vi "Chute.vi"() -> ()   [LabVIEW 2019]
uses:
  <vilib>/Rock Robotics/WPI/ThirdParty/Phoenix-LabVIEW/Motor Controller/Controls/CTRE_Phoenix_MotorControl_ControlMode.ctl
  <vilib>/Rock Robotics/WPI/Solenoid/WPI_SolenoidValue.ctl
  <vilib>/Rock Robotics/WPI/Utilities/WPI_GetSetVariantRefNum.vi
  <vilib>/Rock Robotics/WPI/Solenoid/WPI_SolenoidSetEnum.vi
  <vilib>/Rock Robotics/Network Tables/NT Write Boolean Array.vi
panel:
  in  "Control Mode 4":T1 items=["PercentOutput"=0, "Position"=1, "Velocity"=2, "Current"=3, "Follower"=5, "MotionProfile"=6, "MotionMagic"=7, "MotionProfileArc"=10, "Disabled"=15]
  in  "Control Mode 3":T1 items=["PercentOutput"=0, "Position"=1, "Velocity"=2, "Current"=3, "Follower"=5, "MotionProfile"=6, "MotionMagic"=7, "MotionProfileArc"=10, "Disabled"=15]
  in  "Control Mode 2":T1 items=["PercentOutput"=0, "Position"=1, "Velocity"=2, "Current"=3, "Follower"=5, "MotionProfile"=6, "MotionMagic"=7, "MotionProfileArc"=10, "Disabled"=15]
  in  "Control Mode":T1 items=["PercentOutput"=0, "Position"=1, "Velocity"=2, "Current"=3, "Follower"=5, "MotionProfile"=6, "MotionMagic"=7, "MotionProfileArc"=10, "Disabled"=15]
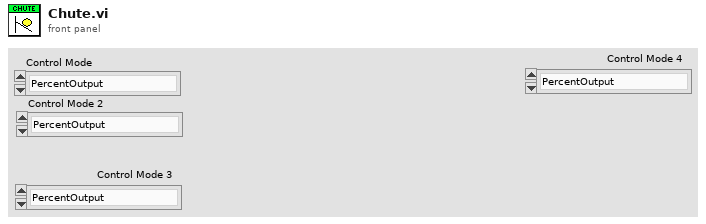
[diagram p1: front panel]
types:
  T1 = typedef "CTRE_Phoenix_MotorControl_ControlMode.ctl" = u16
  T2 = typedef "WPI_JoystickDevRef.ctl" = cluster{"Device":T3}
  T3 = typedef "WPI_JoystickDeviceEnum.ctl" = enum16{"USB 0", "USB 1", "USB 2", "USB 3", "USB 4", "USB 5"}
  T4 = typedef "WPI_SolenoidValue.ctl" = enum16{"Off", "On", "Forward", "Reverse"}
  T5 = typedef "WPI_SolenoidDevRef.ctl" = cluster{"DevStatus":errorcluster, "Pneumatics Control Module":u8, "Forward Solenoid Channel":T6, "Reverse Solenoid Channel":T6}
  T6 = typedef "WPI_SolenoidChannel.ctl" = enum8{"Solenoid 0", "Solenoid 1", "Solenoid 2", "Solenoid 3", "Solenoid 4", "Solenoid 5", "Solenoid 6", "Solenoid 7", "Invalid"}
  T7 = typedef "WPI_MotorControlDeviceRef.ctl" = cluster{"DeviceStatus":errorcluster, "Type":T8, "PWM":cluster{"PWM Channel":T9, "DeadBand":T10}, "CAN":cluster{"Device Number":u8, "SetOutput VI Ref":variant, "GetOutput VI Ref":variant, "Enable VI Ref":variant, "Disable VI Ref":variant, "Data":variant}, "Invert":bool, "DIO PWM":cluster{"PWM \"Enable\" Channel":T9, "DIOChannel":T11, "PWM Rate":dbl}}
  T8 = typedef "WPI_MotorControlType.ctl" = enum16{"PWM", "CAN", "DIO PWM"}
  T9 = typedef "FPGA_DIOPWMChannel.ctl" = enum8{"PWM 0", "PWM 1", "PWM 2", "PWM 3", "PWM 4", "PWM 5", "PWM 6", "PWM 7", "PWM 8", "PWM 9", "PWM MXP 0", "PWM MXP 1", "PWM MXP 2", "PWM MXP 3", "PWM MXP 4", "PWM MXP 5", "PWM MXP 6", "PWM MXP 7", "PWM MXP 8", "PWM MXP 9", "Invalid"}
  T10 = typedef "WPI_PWMDeadband.ctl" = cluster{"Name":string, "maxPositivePwm":i32, "minPositivePwm":i32, "centerPwm":i32, "maxNegativePwm":i32, "minNegativePwm":i32, "angularRange":u16}
  T11 = typedef "FPGA_DIOChannel.ctl" = enum8{"DIO 0", "DIO 1", "DIO 2", "DIO 3", "DIO 4", "DIO 5", "DIO 6", "DIO 7", "DIO 8", "DIO 9", "DIO MXP 0", "DIO MXP 1", "DIO MXP 2", "DIO MXP 3", "DIO MXP 4", "DIO MXP 5", "DIO MXP 6", "DIO MXP 7", "DIO MXP 8", "DIO MXP 9", "DIO MXP 10", "DIO MXP 11", "DIO MXP 12", "DIO MXP 13", "DIO MXP 14", "DIO MXP 15", "SPI Port CS1", "SPI Port CS2", "SPI Port CS3", "SPI Port MISO", "SPI Port MOSI", "Invalid"}
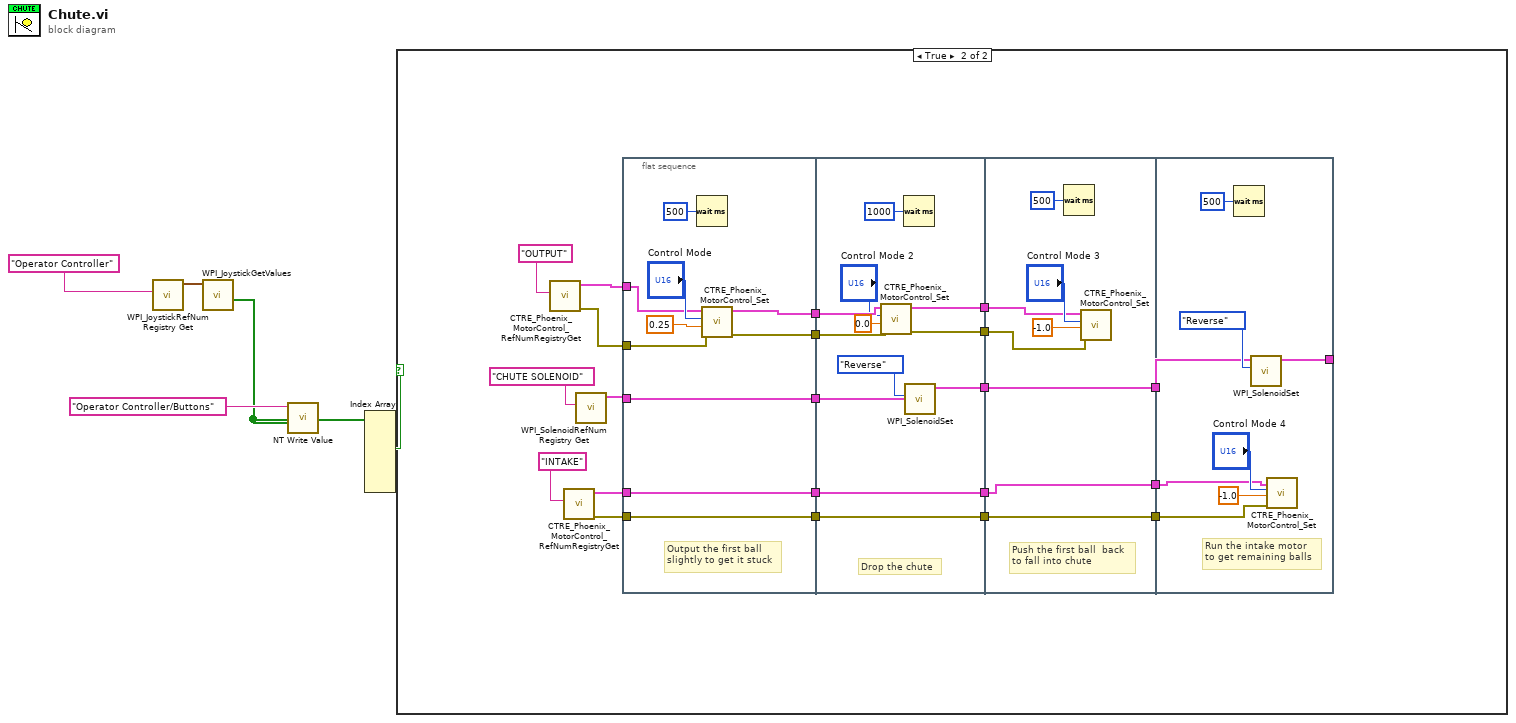
[diagram p0: block diagram]
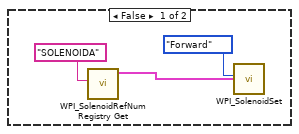
[diagram p2: hidden frame]
diagram:
  n1 = call <vilib>:"WPI_JoystickRefNum Registry Get.vi"("refnum name"="Operator Controller") -> ("JoystickDevRef"=w4:T2)  [unwired: 1 in, 9 out]
  n2 = call <vilib>:"WPI_JoystickGetValues.vi"("JoystickDevRef"=w4) -> ("Buttons"=w2:bool[])  [unwired: 6 in, 4 out]
  n3 = call-poly <vilib>:"NT Write Value.vi"("Boolean Array"=w2, "Name"="Operator Controller/Buttons") -> ()  [unwired: 9 in, 1 out]
  n4 = Index Array(array=w2) -> (element #3=w1:bool)  [unwired: 8 in, 7 out]
  n5 = case shown="True" w1 {
    frame False {
      n6 = call <vilib>:"WPI_SolenoidRefNum Registry Get.vi"("refnum name"="SOLENOIDA") -> ("SolenoidDevRef"=w6:T5)  [unwired: 9 in, 1 out]
      n7 = call-poly <vilib>:"WPI_SolenoidSet.vi"("Value"=WPI_SolenoidValue."Forward", "SolenoidDevRef"=w6) -> ()  [unwired: 8 in, 2 out]
    }
    frame True {
      n8 = call <vilib>:"CTRE_Phoenix_MotorControl_RefNumRegistryGet.vi"("refnum name"="OUTPUT") -> ("error out"=w20:errorcluster, "PhoenixMotorControlDevRef"=w22:T7)  [unwired: 9 in]
      n9 = call <vilib>:"CTRE_Phoenix_MotorControl_RefNumRegistryGet.vi"("refnum name"="INTAKE") -> ("error out"=w12:errorcluster, "PhoenixMotorControlDevRef"=w15:T7)  [unwired: 9 in]
      n10 = call <vilib>:"WPI_SolenoidRefNum Registry Get.vi"("refnum name"="CHUTE SOLENOID") -> ("SolenoidDevRef"=w19:T5)  [unwired: 9 in, 1 out]
      n11 = flat-sequence {
        tunnel: w22 -> [w37]
        tunnel: [w35] -> w29
        tunnel: w20 -> [w34]
        tunnel: [w33] -> w28
        tunnel: [w32] -> w27
        tunnel: w19 -> [w32]
        tunnel: [w31] -> w16
        tunnel: w15 -> [w31]
        tunnel: [w30] -> w13
        tunnel: w12 -> [w30]
        tunnel: w29 -> [w50]
        tunnel: w28 -> [w47]
        tunnel: w27 -> [w45]
        tunnel: [w44] -> w26
        tunnel: [w43] -> w25
        tunnel: [w42] -> w24
        tunnel: [w41] -> w17
        tunnel: w16 -> [w41]
        tunnel: [w40] -> w14
        tunnel: w13 -> [w40]
        tunnel: w24 -> [w59]
        tunnel: w25 -> [w55]
        tunnel: w26 -> [w56]
        tunnel: w17 -> [w53]
        tunnel: w14 -> [w52]
        tunnel: [w59] -> w11
        tunnel: [w53] -> w10
        tunnel: [w52] -> w9
        tunnel: w11 -> [w61]
        tunnel: w10 -> [w64]
        tunnel: w9 -> [w66]
        tunnel: [w60] -> _
        frame #0 {
          # "Output the first ball \nslightly to get it stuck"
          n12 = Wait (ms)(milliseconds to wait=u32 500) -> ()  [unwired: 1 out]
          n13 = call <vilib>:"CTRE_Phoenix_MotorControl_Set.vi"("error in (no error)"=w34, "Output"=0.25, "Control Mode"="Control Mode", "PhoenixMotorControlDevRef"=w37) -> ("error out"=w33:errorcluster, "PhoenixMotorControlDevRef"=w35:T7)  [unwired: 6 in]
        }
        frame #1 {
          # "Drop the chute"
          n14 = call <vilib>:"CTRE_Phoenix_MotorControl_Set.vi"("error in (no error)"=w47, "Output"=0.0, "Control Mode"="Control Mode 2", "PhoenixMotorControlDevRef"=w50) -> ("error out"=w44:errorcluster, "PhoenixMotorControlDevRef"=w43:T7)  [unwired: 6 in]
          n15 = Wait (ms)(milliseconds to wait=u32 1000) -> ()  [unwired: 1 out]
          n16 = call-poly <vilib>:"WPI_SolenoidSet.vi"("Value"=WPI_SolenoidValue."Reverse", "SolenoidDevRef"=w45) -> ("SolenoidDevRef"=w42:T5)  [unwired: 8 in, 1 out]
        }
        frame #2 {
          # "Push the first ball  back\nto fall into chute"
          n17 = Wait (ms)(milliseconds to wait=u32 500) -> ()  [unwired: 1 out]
          n18 = call <vilib>:"CTRE_Phoenix_MotorControl_Set.vi"("error in (no error)"=w56, "Output"=-1.0, "Control Mode"="Control Mode 3", "PhoenixMotorControlDevRef"=w55) -> ()  [unwired: 6 in, 2 out]
        }
        frame #3 {
          # "Run the intake motor\nto get remaining balls"
          n19 = Wait (ms)(milliseconds to wait=u32 500) -> ()  [unwired: 1 out]
          n20 = call-poly <vilib>:"WPI_SolenoidSet.vi"("Value"=WPI_SolenoidValue."Reverse", "SolenoidDevRef"=w61) -> ("SolenoidDevRef"=w60:T5)  [unwired: 8 in, 1 out]
          n21 = call <vilib>:"CTRE_Phoenix_MotorControl_Set.vi"("error in (no error)"=w66, "Output"=-1.0, "Control Mode"="Control Mode 4", "PhoenixMotorControlDevRef"=w64) -> ()  [unwired: 6 in, 2 out]
        }
      }
    }
  }
